vi "Validate Choice-new.vi"(8 "error in (no error)":errorcluster, 10 "Choice":T1, 11 "Reversi in":refnum<class "Reversi.lvclass">) -> (0 "error out":errorcluster, 3 "Reversi out":refnum<class "Reversi.lvclass">)   [LabVIEW 2021]
uses:
  E:/Programs/LabVIEW/Other Stuff/SummerOfLabview/2024/3. Reversi/0. Exploration/OOP/Reversi/Reversi.lvclass
  E:/Programs/LabVIEW/Other Stuff/SummerOfLabview/2024/3. Reversi/0. Exploration/OOP/Reversi/Space Ring.ctl
  E:/Programs/LabVIEW/Other Stuff/SummerOfLabview/2024/3. Reversi/0. Exploration/OOP/Reversi/Space Coordinates.ctl
  E:/Programs/LabVIEW/Other Stuff/SummerOfLabview/2024/3. Reversi/0. Exploration/OOP/Reversi/Space Cluster.ctl
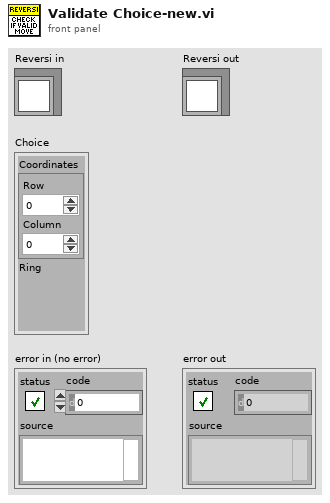
[diagram p1: front panel]
types:
  T1 = typedef "Reversi.lvlib/Reversi.lvclass/Space Cluster.ctl" = cluster{"Coordinates":T2, "Ring":T3}
  T2 = typedef "Reversi.lvlib/Reversi.lvclass/Space Coordinates.ctl" = cluster{"Row":i32, "Column":i32}
  T3 = typedef "Reversi.lvlib/Reversi.lvclass/Space Ring.ctl" = u16
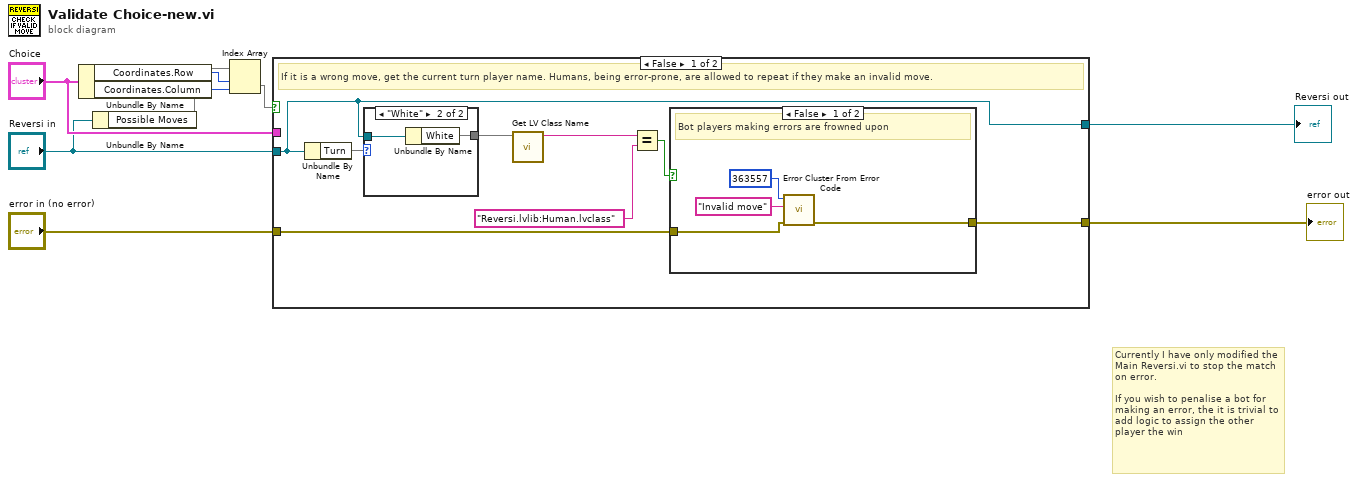
[diagram p0: block diagram]
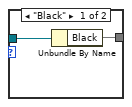
[diagram p2: hidden frame]
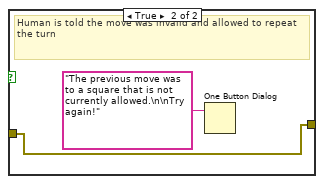
[diagram p3: hidden frame]
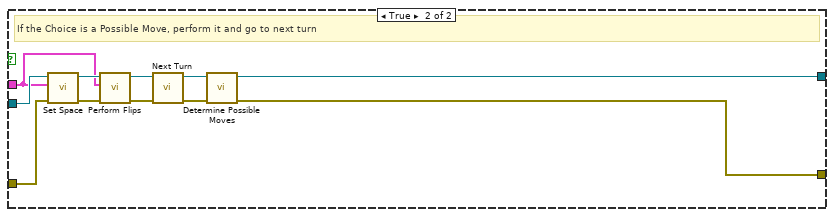
[diagram p4: hidden frame]
diagram:
  # "Currently I have only modified the Main Reversi.vi to stop the match on error.\n\nIf you wish to penalise a bot for making an error, the it is trivial to add logic to assign the other player the win"
  n1 = Unbundle By Name("Choice") -> ("Coordinates.Row"=w8:i32, "Coordinates.Column"=w7:i32)
  n2 = Unbundle By Name("Reversi in") -> ("Possible Moves"=w9)
  n3 = Index Array(array=w9, index (row)=w8, index (col)=w7) -> (element=w6)
  n4 = case shown="False" w6 {
    tunnel: [w13 w28] -> w2
    tunnel: "Reversi in" -> [w13 w38]
    tunnel: "error in (no error)" -> [w11 w37]
    tunnel: [w10 w30] -> w3
    tunnel: "Choice" -> [_ w34]
    frame False {
      # "If it is a wrong move, get the current turn player name. Humans, being error-prone, are allowed to repeat if they make an invalid move."
      n5 = Unbundle By Name(w13) -> ("Turn"=w14)
      n6 = case shown="\"White\"" w14 {
        tunnel: w13 -> [w19 w21]
        tunnel: [w18 w20] -> w12
        frame "Black" {
          n7 = Unbundle By Name(w19) -> ("Black"=w18)
        }
        frame "White" {
          n8 = Unbundle By Name(w21) -> ("White"=w20)
        }
      }
      n9 = call <vilib>:"Get LV Class Name.vi"("object"=w12) -> ("class name"=w17:string)  [unwired: 9 in, 1 out]
      n10 = Equal?(x=w17, y="Reversi.lvlib:Human.lvclass") -> (x = y?=w15:bool)
      n11 = case shown="False" w15 {
        tunnel: w11 -> [w25 w26]
        tunnel: [w24 w26] -> w10
        frame False {
          # "Bot players making errors are frowned upon"
          n12 = call <vilib>:"Error Cluster From Error Code.vi"("error in (no error)"=w25, "error message (\"\")"="Invalid move" ("error message (\"\")"), "error code (0)"=363557) -> ("error out"=w24:errorcluster)  [unwired: 6 in]
        }
        frame True {
          # "Human is told the move was invalid and allowed to repeat the turn"
          n13 = One Button Dialog(message="The previous move was to a square that is not currently allowed.\n\nTry again!") -> ()  [unwired: 1 in, 1 out]
        }
      }
    }
    frame True {
      # "If the Choice is a Possible Move, perform it and go to next turn"
      n14 = call "Set Space.vi"("error in (no error)"=w37, "Space"=w34, "Reversi in"=w38) -> ("error out"=w35:errorcluster, "Reversi out"=w36:refnum<class "Reversi.lvclass">)  [unwired: 7 in]
      n15 = call "Perform Flips.vi"("error in (no error)"=w35, "Choice"=w34, "Reversi in"=w36) -> ("error out"=w33:errorcluster, "Reversi out"=w31:refnum<class "Reversi.lvclass">)  [unwired: 7 in]
      n16 = call "Next Turn.vi"("error in (no error)"=w33, "Reversi in"=w31) -> ("error out"=w32:errorcluster, "Reversi out"=w29:refnum<class "Reversi.lvclass">)  [unwired: 8 in]
      n17 = call "Determine Possible Moves.vi"("error in (no error)"=w32, "Reversi in"=w29) -> ("error out"=w30:errorcluster, "Reversi out"=w28:refnum<class "Reversi.lvclass">)  [unwired: 8 in]
    }
  }
  "error out" <- w3
  "Reversi out" <- w2
